vi "UPRcontroller_v00_basedonlsmv66.vi"() -> ()   [LabVIEW 2015] (continued)
                n2507 = property on="srateAODOtt" class="DigNum (strict)"("Visible"=TRUE, "DisabledEnum"=T8."Enabled" ("Disabled")) -> ()  [unwired: 2 in, 2 out]
                n2508 = call "2pparameters.vi"("command"="get") -> ("params out"=w5803:T12)  [unwired: 1 in]
                n2509 = Bundle By Name(cluster=w5803, "type"="Timetrace") -> (w5797:T12)
                n2510 = call "2pparameters.vi"("Params in"=w5797, "command"="set") -> ()  [unwired: 1 out]
                n2511 = property on="Sampling rate" class="DigNum (strict)"("Visible"=FALSE, "DisabledEnum"=T8."Disabled" ("Disabled")) -> ()  [unwired: 2 in, 2 out]
              }
            }
          }
          event "Laserpower  (%)": Value Change {
            n2512 = event-data() -> ("OldVal"=w5832:dbl, "NewVal"=w5833:dbl)  [unwired: 1 in, 4 out]
            n2513 = Not Equal?(x=w5832, y=w5833) -> (x != y?=w5834:bool)
            n2514 = case shown="True" w5834 {
              tunnel: w5833 -> [_ w5836]
              frame False {
              }
              frame True {
                n2515 = local read "wavelength(nm)"() -> (w5837:dbl)
                n2516 = call "configuration.vi"("command"="get") -> ("config out"=w5841:T14)  [unwired: 2 in, 1 out]
                n2517 = call "pockelscellcalibration.vi"("l"=w5837, "T"=w5836) -> ("Vout"=w5835:dbl)
                n2518 = Unbundle By Name(w5841) -> ("Vto2P"=w5840:i32, "AOlines"=w5839:tag[])
                n2519 = property on="lpow" class="DigNum (strict)"("Value"=w5836) -> ()  [unwired: 2 in, 2 out]
                n2520 = local write "Vpockels"(w5835) -> ()
                n2521 = Index Array(array=w5839, index=w5840) -> (element=w5838:tag)
                n2522 = call-poly <vilib>:"DAQmx Create Virtual Channel.vi"("physical channels"=w5838) -> ("task out"=w5844:refnum<k21>, "error out"=w5843:errorcluster)  [unwired: 13 in]
                n2523 = call-poly <vilib>:"DAQmx Write.vi"("task/channels in"=w5844, "data"=w5835, "error in"=w5843) -> ("task out"=w5845:refnum<k21>, "error out"=w5846:errorcluster)  [unwired: 10 in, 1 out]
                n2524 = call <vilib>:"DAQmx Start Task.vi"("task/channels in"=w5845, "error in"=w5846) -> ("task out"=w5847:refnum<k21>, "error out"=w5848:errorcluster)  [unwired: 12 in]
                n2525 = call <vilib>:"DAQmx Stop Task.vi"("task/channels in"=w5847, "error in"=w5848) -> ("task out"=w5849:refnum<k21>, "error out"=w5850:errorcluster)  [unwired: 12 in]
                n2526 = call <vilib>:"DAQmx Clear Task.vi"("task in"=w5849, "error in"=w5850) -> ()  [unwired: 13 in, 1 out]
              }
            }
          }
          event "lpow": Value Change {
            n2527 = event-data() -> ("OldVal"=w5851:dbl, "NewVal"=w5852:dbl)  [unwired: 1 in, 4 out]
            n2528 = Not Equal?(x=w5851, y=w5852) -> (x != y?=w5853:bool)
            n2529 = case shown="True" w5853 {
              tunnel: w5852 -> [_ w5856]
              frame False {
              }
              frame True {
                n2530 = local read "wavelength(nm)"() -> (w5855:dbl)
                n2531 = call "pockelscellcalibration.vi"("l"=w5855, "T"=w5856) -> ("Vout"=w5854:dbl)
                n2532 = call "configuration.vi"("command"="get") -> ("config out"=w5860:T14)  [unwired: 2 in, 1 out]
                n2533 = Unbundle By Name(w5860) -> ("Vto2P"=w5859:i32, "AOlines"=w5858:tag[])
                n2534 = local write "Vpockels"(w5854) -> ()
                n2535 = property on="Laserpower  (%)" class="Slide (strict)"("Value"=w5856) -> ()  [unwired: 2 in, 2 out]
                n2536 = Index Array(array=w5858, index=w5859) -> (element=w5857:tag)
                n2537 = call-poly <vilib>:"DAQmx Create Virtual Channel.vi"("physical channels"=w5857) -> ("task out"=w5863:refnum<k21>, "error out"=w5862:errorcluster)  [unwired: 13 in]
                n2538 = call-poly <vilib>:"DAQmx Write.vi"("task/channels in"=w5863, "data"=w5854, "error in"=w5862) -> ("task out"=w5864:refnum<k21>, "error out"=w5865:errorcluster)  [unwired: 10 in, 1 out]
                n2539 = call <vilib>:"DAQmx Start Task.vi"("task/channels in"=w5864, "error in"=w5865) -> ("task out"=w5866:refnum<k21>, "error out"=w5867:errorcluster)  [unwired: 12 in]
                n2540 = call <vilib>:"DAQmx Stop Task.vi"("task/channels in"=w5866, "error in"=w5867) -> ("task out"=w5868:refnum<k21>, "error out"=w5869:errorcluster)  [unwired: 12 in]
                n2541 = call <vilib>:"DAQmx Clear Task.vi"("task in"=w5868, "error in"=w5869) -> ()  [unwired: 13 in, 1 out]
              }
            }
          }
          event "sealtest": Value Change {
            n2542 = event-data() -> ()  [unwired: 1 in, 6 out]
            n2543 = case shown="True" "sealtest" {
              frame False {
              }
              frame True {
                n2544 = stacked-sequence {
                  seq-local: [w5871 _ _ _ _ _ _] -> [_ w5906 _ w5958 _ _ _]
                  frame #0 {
                    n2545 = stacked-sequence {
                      tunnel: [_ w5885 _] -> w5871
                      frame #0 {
                        n2546 = call "2pparameters.vi"("command"="get") -> ("params out"=w5877:T12)  [unwired: 1 in]
                        n2547 = Unbundle By Name(w5877) -> ("autoshutter"=w5878:bool, "aAS"=w5872:u32[])
                        n2548 = local read "OCchecked?"() -> (w5875:bool)
                        n2549 = call "sealtestwfparams.vi"("command"="set") -> ()  [unwired: 6 in, 1 out]
                        n2550 = case shown="False" w5875 {
                          frame False {
                            n2551 = One Button Dialog(message="Is the OC gain correct?", button name ("OK")="ok") -> (true=w5879:bool)
                            n2552 = local write "OCchecked?"(w5879) -> ()
                          }
                          frame True {
                          }
                        }
                        n2553 = case shown="True" w5878 {
                          tunnel: w5872 -> [_ w5882]
                          frame False {
                          }
                          frame True {
                            n2554 = call "shuttercontrol_multi.vi"("Autoshutter Chans"=w5882, "command"="close") -> ()  [unwired: 1 in, 1 out]
                          }
                        }
                        n2555 = call "allAI-temp.vi"("command"=enum16{"get", "set", "clear", "append"}."clear") -> ()  [unwired: 3 in, 2 out]
                      }
                      frame #1 {
                        n2556 = call "sealtestwfparams.vi"("command"="get") -> ("Params out"=w5891:T25)  [unwired: 6 in]
                        n2557 = Unbundle By Name(w5891) -> ("AO parameters"=w5889:T26)
                        n2558 = Index Array(array=w5889, index=0) -> (element=w5888:T27)
                        n2559 = call "generateRampedSquareWave_fromAOparameters.vi"("AO params"=w5888) -> ("Waveform"=w5884:waveform(dbl), "wflength"=w5885:i32)
                        n2560 = Build Array(w5884) -> (w5887:waveform(dbl)[])
                        n2561 = call "waveformssealtestbuffer.vi"("AO wf in"=w5887, "command"="set") -> ()  [unwired: 1 out]
                      }
                      frame #2 {
                        n2562 = local read "Vholding (mV)"() -> (w5894:sgl)
                        n2563 = local read "Current Clamp"() -> (w5900:bool)
                        n2564 = local read "Voltage Clamp"() -> (w5899:bool)
                        n2565 = local read "OCgain"() -> (w5895:sgl)
                        n2566 = local read "CC_ICgain"() -> (w5898:dbl)
                        n2567 = local read "holdon"() -> (w5893:bool)
                        n2568 = call "patchparameters.vi"("command"="get") -> ("Params out"=w5902:T16)  [unwired: 1 in]
                        n2569 = Bundle By Name(cluster=w5902, "VC"=w5899, "CC"=w5900, "CC_icg (pA/mv)"=w5898, "VC_icg (mV/mV)"=10.0, "OCG (mV/pA)"=w5895, "OVG (mV/mV)"=0.1, "Vhold (mV)"=w5894, "holdon"=w5893) -> (w5901:T16)
                        n2570 = call "patchparameters.vi"("Params in"=w5901, "command"="set") -> ()  [unwired: 1 out]
                      }
                    }
                  }
                  frame #1 {
                    w5905 = 2
                    n2571 = call "patchparameters.vi"("command"="get") -> ("Params out"=w5913:T16)  [unwired: 1 in]
                    n2572 = Unbundle By Name(w5913) -> ("holdon"=w5912:bool, "Vhold (mV)"=w5911:sgl, "CC_icg (pA/mv)"=w5919:sgl, "CC"=w5917:bool, "VC_icg (mV/mV)"=w5918:sgl)
                    n2573 = Select(t=w5919, s=w5917, f=w5918) -> (s? t:f=w5920:sgl)
                    n2574 = To Single Precision Float(number=0.001 ("y")) -> (single precision float=w5921:sgl)
                    n2575 = Compound Arithmetic op=MULTIPLY(w5911, w5920, w5921) -> (w5915:sgl)
                    n2576 = case shown="False" w5912 {
                      tunnel: w5915 -> [_ w5933]
                      tunnel: [0.0 w5933] -> w5908
                      frame False {
                      }
                      frame True {
                      }
                    }
                    n2577 = Greater Than 0?(x=w5905) -> (x > 0?=w5907:bool)
                    n2578 = case shown="True" w5907 {
                      tunnel: w5906 -> [_ w5922]
                      tunnel: w5905 -> [_ w5925]
                      frame False {
                      }
                      frame True {
                        n2579 = Initialize Array(sgl 0.0 ("element"), w5925, w5922) -> (w5923:sgl[][])
                        n2580 = call "allAI-temp.vi"("array in"=w5923, "command"=enum16{"get", "set", "clear", "append"}."set") -> ()  [unwired: 2 in, 2 out]
                      }
                    }
                    n2581 = flat-sequence {
                      tunnel: w5906 -> [w5929]
                      tunnel: w5906 -> [w5928]
                      tunnel: [w5928] -> w5910
                      tunnel: [w5927] -> w5909
                      tunnel: w5908 -> [w5927]
                      tunnel: w5910 -> [w5931]
                      tunnel: w5909 -> [w5930]
                      frame #0 {
                        n2582 = call "prepAI_sealtest.vi"("samples per channel"=w5929) -> ()  [unwired: 2 in]
                      }
                      frame #1 {
                        n2583 = call "prepAO_sealtest.vi"("Vhold"=w5930, "samples per channel"=w5931) -> ()  [unwired: 1 in]
                      }
                    }
                  }
                  frame #2 {
                    n2584 = stacked-sequence {
                      frame #0 {
                        n2585 = call "tempconfigAO_seal.vi"("command"="get") -> ("Temp Config out"=w5937:T28)  [unwired: 1 in]
                        n2586 = Unbundle By Name(w5937) -> ("AO"=w5938:refnum<k21>[], "E_AO"=w5939:errorcluster[])
                        n2587 = for {
                          tunnel: w5938 -> [w5947] mode=indexing
                          tunnel: w5939 -> [w5946] mode=indexing
                          tunnel: [w5945] -> w5941 mode=indexing
                          tunnel: [w5944] -> w5942 mode=indexing
                          n2588 = call <vilib>:"DAQmx Start Task.vi"("task/channels in"=w5947, "error in"=w5946) -> ("task out"=w5945:refnum<k21>, "error out"=w5944:errorcluster)  [unwired: 12 in]
                        }
                        n2589 = call "tempconfigAO_seal.vi"("command"="get") -> ("Temp Config out"=w5940:T28)  [unwired: 1 in]
                        n2590 = Bundle By Name(cluster=w5940, "AO"=w5941, "E_AO"=w5942) -> (w5943:T28)
                        n2591 = call "tempconfigAO_seal.vi"("Temp Config in"=w5943, "command"="set") -> ()  [unwired: 1 out]
                      }
                      frame #1 {
                        n2592 = call "tempconfigAI_seal.vi"("command"="get") -> ("Temp Config out"=w5949:T29)  [unwired: 1 in]
                        n2593 = Unbundle By Name(w5949) -> ("AI"=w5954:refnum<k21>, "E_AI"=w5955:errorcluster)
                        n2594 = call <vilib>:"DAQmx Start Task.vi"("task/channels in"=w5954, "error in"=w5955) -> ("task out"=w5956:refnum<k21>, "error out"=w5957:errorcluster)  [unwired: 12 in]
                        n2595 = call "tempconfigAI_seal.vi"("command"="get") -> ("Temp Config out"=w5951:T29)  [unwired: 1 in]
                        n2596 = Bundle By Name(cluster=w5951, "AI"=w5956, "E_AI"=w5957) -> (w5953:T29)
                        n2597 = call "tempconfigAI_seal.vi"("Temp Config in"=w5953, "command"="set") -> ()  [unwired: 1 out]
                      }
                    }
                  }
                  frame #3 {
                    n2598 = while {
                      tunnel: w5958 -> [w5959]
                      stop <- w5960 stop-if-true
                      n2599 = stacked-sequence {
                        seq-local: [_ _ _ w6001 _ _] -> [_ _ _ _ w6053 _]
                        seq-local: [w5962 _ _ _ _ _] -> [_ w5971 _ w5994 w6042 w6073]
                        tunnel: w5959 -> [_ _ w5979 _ w6041 _]
                        frame #0 {
                          n2600 = call "patchparameters.vi"("command"="get") -> ("Params out"=w5969:T16)  [unwired: 1 in]
                          n2601 = local read "Vholding (mV)"() -> (w5966:sgl)
                          n2602 = Unbundle By Name(w5969) -> ("Vhold (mV)"=w5965:sgl, "holdon"=w5968:bool)
                          n2603 = local read "holdon"() -> (w5967:bool)
                          n2604 = Not Equal?(x=w5966, y=w5965) -> (x != y?=w5964:bool)
                          n2605 = Not Equal?(x=w5968, y=w5967) -> (x != y?=w5963:bool)
                          n2606 = Or(x=w5964, y=w5963) -> (x .or. y?=w5962:bool)
                        }
                        frame #1 {
                          n2607 = case shown="True" w5971 {
                            frame False {
                            }
                            frame True {
                              n2608 = local read "Vholding (mV)"() -> (w5974:sgl)
                              n2609 = local read "holdon"() -> (w5972:bool)
                              n2610 = call "patchparameters.vi"("command"="get") -> ("Params out"=w5975:T16)  [unwired: 1 in]
                              n2611 = Bundle By Name(cluster=w5975, "Vhold (mV)"=w5974, "holdon"=w5972) -> (w5973:T16)
                              n2612 = call "patchparameters.vi"("Params in"=w5973, "command"="set") -> ()  [unwired: 1 out]
                            }
                          }
                        }
                        frame #2 {
                          n2613 = call "tempconfigAI_seal.vi"("command"="get") -> ("Temp Config out"=w5989:T29)  [unwired: 1 in]
                          n2614 = Unbundle By Name(w5989) -> ("AI"=w5988:refnum<k21>, "E_AI"=w5987:errorcluster)
                          n2615 = call-poly <vilib>:"DAQmx Read.vi"("task/channels in"=w5988, "number of samples per channel"=w5979, "timeout"=10.0, "error in"=w5987) -> ("task out"=w5983:refnum<k21>, "data"=w5980:i16[][], "error out"=w5992:errorcluster)  [unwired: 9 in]
                          n2616 = call "tempconfigAI_seal.vi"("command"="get") -> ("Temp Config out"=w5984:T29)  [unwired: 1 in]
                          n2617 = Bundle By Name(cluster=w5984, "AI"=w5983, "E_AI"=w5992) -> (w5991:T29)
                          n2618 = To Single Precision Float(number=w5980) -> (single precision float=w5982:sgl[][])
                          n2619 = call "tempconfigAI_seal.vi"("Temp Config in"=w5991, "command"="set") -> ()  [unwired: 1 out]
                          n2620 = call "allAI-temp.vi"("array in"=w5982, "command"=enum16{"get", "set", "clear", "append"}."set") -> ()  [unwired: 2 in, 2 out]
                        }
                        frame #3 {
                          n2621 = case shown="True" w5994 {
                            frame False {
                            }
                            frame True {
                              n2622 = call "tempconfigAO_seal.vi"("command"="get") -> ("Temp Config out"=w6030:T28)  [unwired: 1 in]
                              n2623 = Unbundle By Name(w6030) -> ("AO"=w6029:refnum<k21>[], "E_AO"=w6028:errorcluster[])
                              n2624 = call "tempconfigAI_seal.vi"("command"="get") -> ("Temp Config out"=w6017:T29)  [unwired: 1 in]
                              n2625 = Unbundle By Name(w6017) -> ("AI"=w6018:refnum<k21>, "E_AI"=w6019:errorcluster)
                              n2626 = for {
                                tunnel: w6029 -> [w6034] mode=indexing
                                tunnel: w6028 -> [w6033] mode=indexing
                                tunnel: [w6032] -> w6024 mode=indexing
                                n2627 = call <vilib>:"DAQmx Stop Task.vi"("task/channels in"=w6034, "error in"=w6033) -> ("task out"=w6035:refnum<k21>, "error out"=w6036:errorcluster)  [unwired: 12 in]
                                n2628 = call <vilib>:"DAQmx Clear Task.vi"("task in"=w6035, "error in"=w6036) -> ("error out"=w6032:errorcluster)  [unwired: 13 in]
                              }
                              n2629 = call <vilib>:"DAQmx Stop Task.vi"("task/channels in"=w6018, "error in"=w6019) -> ("task out"=w6015:refnum<k21>, "error out"=w6014:errorcluster)  [unwired: 12 in]
                              n2630 = call <vilib>:"DAQmx Clear Task.vi"("task in"=w6015, "error in"=w6014) -> ("error out"=w6013:errorcluster)  [unwired: 13 in]
                              n2631 = call "tempconfigAO_seal.vi"("command"="get") -> ("Temp Config out"=w6025:T28)  [unwired: 1 in]
                              n2632 = Bundle By Name(cluster=w6025, "E_AO"=w6024) -> (w6023:T28)
                              n2633 = call "tempconfigAI_seal.vi"("command"="get") -> ("Temp Config out"=w6021:T29)  [unwired: 1 in]
                              n2634 = Bundle By Name(cluster=w6021, "E_AI"=w6013) -> (w6012:T29)
                              n2635 = call "tempconfigAO_seal.vi"("Temp Config in"=w6023, "command"="set") -> ()  [unwired: 1 out]
                              n2636 = call "tempconfigAI_seal.vi"("Temp Config in"=w6012, "command"="set") -> ()  [unwired: 1 out]
                            }
                          }
                          n2637 = call "allAI-temp.vi"("command"=enum16{"get", "set", "clear", "append"}."get") -> ("array out"=w5998:sgl[][])  [unwired: 3 in, 1 out]
                          n2638 = call "tempconfigAI_seal.vi"("command"="get") -> ("Temp Config out"=w6010:T29)  [unwired: 1 in]
                          n2639 = Unbundle By Name(w6010) -> ("header"=w5993:dbl[])
                          n2640 = Index Array(array=w5998, index (row) #1=1 ("index (row)"), index (row) #2=0 ("index (row)")) -> (element #1=w5996:sgl[], element #2=w5995:sgl[])  [unwired: 2 in]
                          n2641 = local read "OCgain"() -> (w6003:sgl)
                          n2642 = call "Unscaledtoscaled.vi"("Unscaled Data"=w5996, "Header Information"=w5993) -> ("Array"=w6008:sgl[])  [unwired: 1 in]
                          n2643 = call "Unscaledtoscaled.vi"("Unscaled Data"=w5995, "Header Information"=w5993) -> ("Array"=w6011:sgl[])  [unwired: 1 in]
                          n2644 = Multiply(x=w6008, y=0.1) -> (x*y=w6005:dbl[])
                          n2645 = Divide(x=w6011, y=w6003) -> (x/y=w6004:sgl[])
                          n2646 = Build Array(w6005, w6004) -> (w6007:dbl[][])
                          n2647 = Multiply(x=w6007, y=1000.0) -> (x*y=w6001:dbl[][])
                          "Patch readout" <- w6001
                        }
                        frame #4 {
                          n2648 = case shown="True" w6042 {
                            tunnel: w6041 -> [_ w6054]
                            frame False {
                            }
                            frame True {
                              n2649 = call "patchparameters.vi"("command"="get") -> ("Params out"=w6058:T16)  [unwired: 1 in]
                              n2650 = Unbundle By Name(w6058) -> ("holdon"=w6057:bool, "Vhold (mV)"=w6056:sgl, "CC_icg (pA/mv)"=w6064:sgl, "CC"=w6062:bool, "VC_icg (mV/mV)"=w6063:sgl)
                              n2651 = Select(t=w6064, s=w6062, f=w6063) -> (s? t:f=w6065:sgl)
                              n2652 = To Single Precision Float(number=0.001 ("y")) -> (single precision float=w6066:sgl)
                              n2653 = Compound Arithmetic op=MULTIPLY(w6056, w6065, w6066) -> (w6060:sgl)
                              n2654 = case shown="True" w6057 {
                                tunnel: w6060 -> [_ w6071]
                                tunnel: [0.0 w6071] -> w6055
                                frame False {
                                }
                                frame True {
                                }
                              }
                              n2655 = flat-sequence {
                                tunnel: w6054 -> [w6067]
                                tunnel: w6055 -> [w6069]
                                tunnel: w6054 -> [w6068]
                                frame #0 {
                                n2656 = call "prepAI_sealtest.vi"("samples per channel"=w6067) -> ()  [unwired: 2 in]
                                }
                                frame #1 {
                                n2657 = call "prepAO_sealtest.vi"("Vhold"=w6069, "samples per channel"=w6068) -> ()  [unwired: 1 in]
                                }
                              }
                            }
                          }
                          n2658 = call "sealtestwfparams.vi"("command"="get") -> ("Params out"=w6047:T25)  [unwired: 6 in]
                          n2659 = Unbundle By Name(w6047) -> ("AO parameters"=w6048:T26)
                          n2660 = Index Array(array=w6048, index=0) -> (element=w6050:T27)
                          n2661 = Unbundle By Name(w6050) -> ("Cycles"=w6045:dbl, "Start amplitude (V)"=w6044:dbl, "Sampling frequency (Hz)"=w6043:dbl)
                          n2662 = local read "fitpoints"() -> (w6051:dbl)
                          n2663 = script code="V=data(1,:);\nI=data(2,:);\ntres=mean(V);\nspc=(nsamp./ncyc);\nV=V(spc+1:end-spc);\nI=I(spc+1:end-spc);\ndV=mean(V(V>tres))-mean(V(V<tres))\nIcyc=reshape(I,[spc ncyc-2]);\nIcyc=Icyc';\nIcyc=mean(Icyc,1);\ndIss=mean(Icyc(floor(spc*0.15):floor(spc/2)-2))-mean(Icyc(spc*0.65:spc-2))\nRm=dV*1e3/dIss;\n[maxi,ind]=max(Icyc);\nIfit=Icyc(ind+1:ind+1+points-1)-0.5*(mean(Icyc(floor(spc*0.15):floor(spc/2)-2))+mean(Icyc(spc*0.65:spc-2)))\nt=(3:points-1+3)./srate*1000;\nt=t';\nIfit=Ifit';\nc=fit(t,Ifit, 'exp1');\ncoeffs=coeffvalues(c);\nIa=coeffs(1);\nRa=dV*1e3./Ia/2;\ntau=-1./coeffs(2);\ncap=tau/Ra*1000;"("data"=w6053, "nsamp"=w6041, "ncyc"=w6045, "maxV"=w6044, "points"=w6051, "srate"=w6043) -> ("cap"=w6040:dbl, "Ra"=w6039:dbl, "Icyc"=w6038:dbl[], "Rm"=w6037:dbl)  [unwired: 1 in, 1 out]
                          n2664 = local read "set as Rp?"() -> (w6052:bool)
                          n2665 = local write "Cmembrane"(w6040) -> ()
                          n2666 = local write "Rmembrane (MOhm)"(w6037) -> ()
                          n2667 = local write "Racces (MOhm)"(w6039) -> ()
                          n2668 = case shown="True" w6052 {
                            tunnel: w6037 -> [_ w6072]
                            frame False {
                            }
                            frame True {
                              n2669 = local write "Rpipette (MOhm)"(w6072) -> ()
                            }
                          }
                          n2670 = local write "Ifit"(w6038) -> ()
                        }
                        frame #5 {
                          n2671 = local read "set as Rp?"() -> (w6074:bool)
                          n2672 = case shown="True" w6073 {
                            frame False {
                            }
                            frame True {
                              n2673 = stacked-sequence {
                                frame #0 {
                                n2674 = call "tempconfigAO_seal.vi"("command"="get") -> ("Temp Config out"=w6081:T28)  [unwired: 1 in]
                                n2675 = Unbundle By Name(w6081) -> ("AO"=w6080:refnum<k21>[], "E_AO"=w6079:errorcluster[])
                                n2676 = for {
                                tunnel: w6080 -> [w6088] mode=indexing
                                tunnel: w6079 -> [w6087] mode=indexing
                                tunnel: [w6086] -> w6077 mode=indexing
                                tunnel: [w6085] -> w6076 mode=indexing
                                n2677 = call <vilib>:"DAQmx Start Task.vi"("task/channels in"=w6088, "error in"=w6087) -> ("task out"=w6086:refnum<k21>, "error out"=w6085:errorcluster)  [unwired: 12 in]
                                }
                                n2678 = call "tempconfigAO_seal.vi"("command"="get") -> ("Temp Config out"=w6078:T28)  [unwired: 1 in]
                                n2679 = Bundle By Name(cluster=w6078, "AO"=w6077, "E_AO"=w6076) -> (w6075:T28)
                                n2680 = call "tempconfigAO_seal.vi"("Temp Config in"=w6075, "command"="set") -> ()  [unwired: 1 out]
                                }
                                frame #1 {
                                n2681 = call "tempconfigAI_seal.vi"("command"="get") -> ("Temp Config out"=w6090:T29)  [unwired: 1 in]
                                n2682 = Unbundle By Name(w6090) -> ("AI"=w6095:refnum<k21>, "E_AI"=w6096:errorcluster)
                                n2683 = call <vilib>:"DAQmx Start Task.vi"("task/channels in"=w6095, "error in"=w6096) -> ("task out"=w6097:refnum<k21>, "error out"=w6098:errorcluster)  [unwired: 12 in]
                                n2684 = call "tempconfigAI_seal.vi"("command"="get") -> ("Temp Config out"=w6092:T29)  [unwired: 1 in]
                                n2685 = Bundle By Name(cluster=w6092, "AI"=w6097, "E_AI"=w6098) -> (w6094:T29)
                                n2686 = call "tempconfigAI_seal.vi"("Temp Config in"=w6094, "command"="set") -> ()  [unwired: 1 out]
                                }
                              }
                            }
                          }
                          n2687 = case shown="True" w6074 {
                            frame False {
                            }
                            frame True {
                              n2688 = local write "set as Rp?"(FALSE ("set as Rp?")) -> ()
                            }
                          }
                        }
                      }
                      n2689 = local read "sealtest"() -> (w5961:bool)
                      n2690 = Not(x=w5961) -> (.not. x?=w5960:bool)
                    }
                  }
                  frame #4 {
                    n2691 = call "tempconfigAO_seal.vi"("command"="get") -> ("Temp Config out"=w6125:T28)  [unwired: 1 in]
                    n2692 = Unbundle By Name(w6125) -> ("AO"=w6124:refnum<k21>[], "E_AO"=w6123:errorcluster[])
                    n2693 = call "tempconfigAI_seal.vi"("command"="get") -> ("Temp Config out"=w6112:T29)  [unwired: 1 in]
                    n2694 = call "configuration.vi"("command"="get") -> ("config out"=w6106:T14)  [unwired: 2 in, 1 out]
                    n2695 = Unbundle By Name(w6112) -> ("AI"=w6113:refnum<k21>, "E_AI"=w6114:errorcluster)
                    n2696 = Unbundle By Name(w6106) -> ("Device 1 sampleclock out"=w6103:tag, "Device 1 Starttrigger out"=w6102:tag)
                    n2697 = for {
                      tunnel: w6124 -> [w6129] mode=indexing
                      tunnel: w6123 -> [w6128] mode=indexing
                      tunnel: [w6127] -> w6119 mode=indexing
                      n2698 = call <vilib>:"DAQmx Stop Task.vi"("task/channels in"=w6129, "error in"=w6128) -> ("task out"=w6130:refnum<k21>, "error out"=w6131:errorcluster)  [unwired: 12 in]
                      n2699 = call <vilib>:"DAQmx Clear Task.vi"("task in"=w6130, "error in"=w6131) -> ("error out"=w6127:errorcluster)  [unwired: 13 in]
                    }
                    n2700 = call <vilib>:"DAQmx Stop Task.vi"("task/channels in"=w6113, "error in"=w6114) -> ("task out"=w6110:refnum<k21>, "error out"=w6109:errorcluster)  [unwired: 12 in]
                    n2701 = call <vilib>:"DAQmx Disconnect Terminals.vi"("source terminal"=tag "/Dev1/ai/SampleClock", "destination terminal"=w6103) -> ("error out"=w6100:errorcluster)  [unwired: 13 in]
                    n2702 = call <vilib>:"DAQmx Clear Task.vi"("task in"=w6110, "error in"=w6109) -> ("error out"=w6108:errorcluster)  [unwired: 13 in]
                    n2703 = call "tempconfigAO_seal.vi"("command"="get") -> ("Temp Config out"=w6120:T28)  [unwired: 1 in]
                    n2704 = Bundle By Name(cluster=w6120, "E_AO"=w6119) -> (w6118:T28)
                    n2705 = call "tempconfigAI_seal.vi"("command"="get") -> ("Temp Config out"=w6116:T29)  [unwired: 1 in]
                    n2706 = Bundle By Name(cluster=w6116, "E_AI"=w6108) -> (w6107:T29)
                    n2707 = call "tempconfigAO_seal.vi"("Temp Config in"=w6118, "command"="set") -> ()  [unwired: 1 out]
                    n2708 = call "tempconfigAI_seal.vi"("Temp Config in"=w6107, "command"="set") -> ()  [unwired: 1 out]
                    n2709 = call <vilib>:"DAQmx Disconnect Terminals.vi"("source terminal"=tag "/Dev1/ai/StartTrigger", "destination terminal"=w6102, "error in"=w6100) -> ()  [unwired: 12 in, 1 out]
                  }
                  frame #5 {
                    n2710 = call "zeropatch.vi"() -> ()  [unwired: 12 in]
                  }
                  frame #6 {
                    w6135 = T24 4 items=["no dialog", "OK message", "continue or stop message", "OK message + warnings", "continue/stop + warnings"] ("type of dialog (OK msg:1)")
                    n2711 = call "displayerrors.vi"() -> ("error IO"=w6134:errorcluster)
                    n2712 = call <vilib>:"Simple Error Handler.vi"("type of dialog (OK msg:1)"=w6135, "error in (no error)"=w6134) -> ("error out"=w6133:errorcluster)  [unwired: 3 in, 4 out]
                    n2713 = call <vilib>:"Clear Errors.vi"("error in (no error)"=w6133) -> ("error out"=w6132:errorcluster)  [unwired: 5 in, 1 out]
                    n2714 = call "seterrors.vi"("error IO"=w6132) -> ()
                  }
                }
              }
            }
          }
          event "readpatch": Value Change {
            n2715 = event-data() -> ()  [unwired: 1 in, 6 out]
            n2716 = local read "readpatch"() -> (w6136:bool)
            n2717 = case shown="True" w6136 {
              frame False {
              }
              frame True {
                n2718 = stacked-sequence {
                  seq-local: [w6137 _ _ _ _ _] -> [_ w6172 _ w6224 _ _]
                  frame #0 {
                    n2719 = stacked-sequence {
                      tunnel: [_ w6151 _] -> w6137
                      frame #0 {
                        n2720 = call "2pparameters.vi"("command"="get") -> ("params out"=w6143:T12)  [unwired: 1 in]
                        n2721 = Unbundle By Name(w6143) -> ("autoshutter"=w6144:bool, "aAS"=w6138:u32[])
                        n2722 = local read "OCchecked?"() -> (w6141:bool)
                        n2723 = call "sealtestwfparams.vi"("command"="set") -> ()  [unwired: 6 in, 1 out]
                        n2724 = case shown="False" w6141 {
                          frame False {
                            n2725 = One Button Dialog(message="Is the OC gain correct?", button name ("OK")="ok") -> (true=w6145:bool)
                            n2726 = local write "OCchecked?"(w6145) -> ()
                          }
                          frame True {
                          }
                        }
                        n2727 = case shown="True" w6144 {
                          tunnel: w6138 -> [_ w6148]
                          frame False {
                          }
                          frame True {
                            n2728 = call "shuttercontrol_multi.vi"("Autoshutter Chans"=w6148, "command"="close") -> ()  [unwired: 1 in, 1 out]
                          }
                        }
                        n2729 = call "allAI-temp.vi"("command"=enum16{"get", "set", "clear", "append"}."clear") -> ()  [unwired: 3 in, 2 out]
                      }
                      frame #1 {
                        n2730 = call "sealtestwfparams.vi"("command"="get") -> ("Params out"=w6157:T25)  [unwired: 6 in]
                        n2731 = Unbundle By Name(w6157) -> ("AO parameters"=w6155:T26)
                        n2732 = Index Array(array=w6155, index=1) -> (element=w6154:T27)
                        n2733 = call "generateRampedSquareWave_fromAOparameters.vi"("AO params"=w6154) -> ("Waveform"=w6150:waveform(dbl), "wflength"=w6151:i32)
                        n2734 = Build Array(w6150) -> (w6153:waveform(dbl)[])
                        n2735 = call "waveformssealtestbuffer.vi"("AO wf in"=w6153, "command"="set") -> ()  [unwired: 1 out]
                      }
                      frame #2 {
                        n2736 = local read "Vholding (mV)"() -> (w6160:sgl)
                        n2737 = local read "Current Clamp"() -> (w6166:bool)
                        n2738 = local read "Voltage Clamp"() -> (w6165:bool)
                        n2739 = local read "OCgain"() -> (w6161:sgl)
                        n2740 = local read "CC_ICgain"() -> (w6164:dbl)
                        n2741 = local read "holdon"() -> (w6159:bool)
                        n2742 = call "patchparameters.vi"("command"="get") -> ("Params out"=w6168:T16)  [unwired: 1 in]
                        n2743 = Bundle By Name(cluster=w6168, "VC"=w6165, "CC"=w6166, "CC_icg (pA/mv)"=w6164, "VC_icg (mV/mV)"=10.0, "OCG (mV/pA)"=w6161, "OVG (mV/mV)"=0.1, "Vhold (mV)"=w6160, "holdon"=w6159) -> (w6167:T16)
                        n2744 = call "patchparameters.vi"("Params in"=w6167, "command"="set") -> ()  [unwired: 1 out]
                      }
                    }
                  }
                  frame #1 {
                    w6171 = 2
                    n2745 = call "patchparameters.vi"("command"="get") -> ("Params out"=w6179:T16)  [unwired: 1 in]
                    n2746 = Unbundle By Name(w6179) -> ("holdon"=w6178:bool, "Vhold (mV)"=w6177:sgl, "CC_icg (pA/mv)"=w6185:sgl, "CC"=w6183:bool, "VC_icg (mV/mV)"=w6184:sgl)
                    n2747 = Select(t=w6185, s=w6183, f=w6184) -> (s? t:f=w6186:sgl)
                    n2748 = To Single Precision Float(number=0.001 ("y")) -> (single precision float=w6187:sgl)
                    n2749 = Compound Arithmetic op=MULTIPLY(w6177, w6186, w6187) -> (w6181:sgl)
                    n2750 = case shown="False" w6178 {
                      tunnel: w6181 -> [_ w6199]
                      tunnel: [0.0 w6199] -> w6174
                      frame False {
                      }
                      frame True {
                      }
                    }
                    n2751 = Greater Than 0?(x=w6171) -> (x > 0?=w6173:bool)
                    n2752 = case shown="True" w6173 {
                      tunnel: w6172 -> [_ w6188]
                      tunnel: w6171 -> [_ w6191]
                      frame False {
                      }
                      frame True {
                        n2753 = Initialize Array(sgl 0.0 ("element"), w6191, w6188) -> (w6189:sgl[][])
                        n2754 = call "allAI-temp.vi"("array in"=w6189, "command"=enum16{"get", "set", "clear", "append"}."set") -> ()  [unwired: 2 in, 2 out]
                      }
                    }
                    n2755 = flat-sequence {
                      tunnel: w6172 -> [w6195]
                      tunnel: w6172 -> [w6194]
                      tunnel: [w6194] -> w6176
                      tunnel: [w6193] -> w6175
                      tunnel: w6174 -> [w6193]
                      tunnel: w6176 -> [w6197]
                      tunnel: w6175 -> [w6196]
                      frame #0 {
                        n2756 = call "prepAI_sealtest.vi"("samples per channel"=w6195) -> ()  [unwired: 2 in]
                      }
                      frame #1 {
                        n2757 = call "prepAO_sealtest.vi"("Vhold"=w6196, "samples per channel"=w6197) -> ()  [unwired: 1 in]
                      }
                    }
                  }
                  frame #2 {
                    n2758 = stacked-sequence {
                      frame #0 {
                        n2759 = call "tempconfigAO.vi"("command"="get") -> ("Temp Config out"=w6203:T28)  [unwired: 1 in]
                        n2760 = Unbundle By Name(w6203) -> ("AO"=w6204:refnum<k21>[], "E_AO"=w6205:errorcluster[])
                        n2761 = for {
                          tunnel: w6204 -> [w6213] mode=indexing
                          tunnel: w6205 -> [w6212] mode=indexing
                          tunnel: [w6211] -> w6207 mode=indexing
                          tunnel: [w6210] -> w6208 mode=indexing
                          n2762 = call <vilib>:"DAQmx Start Task.vi"("task/channels in"=w6213, "error in"=w6212) -> ("task out"=w6211:refnum<k21>, "error out"=w6210:errorcluster)  [unwired: 12 in]
                        }
                        n2763 = call "tempconfigAO.vi"("command"="get") -> ("Temp Config out"=w6206:T28)  [unwired: 1 in]
                        n2764 = Bundle By Name(cluster=w6206, "AO"=w6207, "E_AO"=w6208) -> (w6209:T28)
                        n2765 = call "tempconfigAO.vi"("Temp Config in"=w6209, "command"="set") -> ()  [unwired: 1 out]
                      }
                      frame #1 {
                        n2766 = call "tempconfigAI.vi"("command"="get") -> ("Temp Config out"=w6215:T29)  [unwired: 1 in]
                        n2767 = Unbundle By Name(w6215) -> ("AI"=w6220:refnum<k21>, "E_AI"=w6221:errorcluster)
                        n2768 = call <vilib>:"DAQmx Start Task.vi"("task/channels in"=w6220, "error in"=w6221) -> ("task out"=w6222:refnum<k21>, "error out"=w6223:errorcluster)  [unwired: 12 in]
                        n2769 = call "tempconfigAI.vi"("command"="get") -> ("Temp Config out"=w6217:T29)  [unwired: 1 in]
                        n2770 = Bundle By Name(cluster=w6217, "AI"=w6222, "E_AI"=w6223) -> (w6219:T29)
                        n2771 = call "tempconfigAI.vi"("Temp Config in"=w6219, "command"="set") -> ()  [unwired: 1 out]
                      }
                    }
                  }
                  frame #3 {
                    n2772 = while {
                      tunnel: w6224 -> [w6225]
                      stop <- w6226 stop-if-true
                      n2773 = local read "readpatch"() -> (w6229:bool)
                      n2774 = Not(x=w6229) -> (.not. x?=w6228:bool)
                      n2775 = case shown="False" w6228 {
                        tunnel: w6225 -> [w6230 _]
                        frame False {
                          n2776 = stacked-sequence {
                            seq-local: [w6231 _ _ _ _ _] -> [_ w6240 _ w6263 w6310 w6329]
                            tunnel: w6230 -> [_ _ w6248 _ w6309 _]
                            frame #0 {
                              n2777 = call "patchparameters.vi"("command"="get") -> ("Params out"=w6238:T16)  [unwired: 1 in]
                              n2778 = local read "Vholding (mV)"() -> (w6235:sgl)
                              n2779 = Unbundle By Name(w6238) -> ("Vhold (mV)"=w6234:sgl, "holdon"=w6237:bool)
                              n2780 = local read "holdon"() -> (w6236:bool)
                              n2781 = Not Equal?(x=w6235, y=w6234) -> (x != y?=w6233:bool)
                              n2782 = Not Equal?(x=w6237, y=w6236) -> (x != y?=w6232:bool)
                              n2783 = Or(x=w6233, y=w6232) -> (x .or. y?=w6231:bool)
                            }
                            frame #1 {
                              n2784 = case shown="False" w6240 {
                                frame False {
                                }
                                frame True {
                                n2785 = local read "Vholding (mV)"() -> (w6243:sgl)
                                n2786 = local read "holdon"() -> (w6241:bool)
                                n2787 = call "patchparameters.vi"("command"="get") -> ("Params out"=w6244:T16)  [unwired: 1 in]
                                n2788 = Bundle By Name(cluster=w6244, "Vhold (mV)"=w6243, "holdon"=w6241) -> (w6242:T16)
                                n2789 = call "patchparameters.vi"("Params in"=w6242, "command"="set") -> ()  [unwired: 1 out]
                                }
                              }
                            }
                            frame #2 {
                              n2790 = call "tempconfigAI.vi"("command"="get") -> ("Temp Config out"=w6258:T29)  [unwired: 1 in]
                              n2791 = Unbundle By Name(w6258) -> ("AI"=w6257:refnum<k21>, "E_AI"=w6256:errorcluster)
                              n2792 = call-poly <vilib>:"DAQmx Read.vi"("task/channels in"=w6257, "number of samples per channel"=w6248, "timeout"=10.0, "error in"=w6256) -> ("task out"=w6252:refnum<k21>, "data"=w6249:i16[][], "error out"=w6261:errorcluster)  [unwired: 9 in]
                              n2793 = call "tempconfigAI.vi"("command"="get") -> ("Temp Config out"=w6253:T29)  [unwired: 1 in]
                              n2794 = Bundle By Name(cluster=w6253, "AI"=w6252, "E_AI"=w6261) -> (w6260:T29)
                              n2795 = To Single Precision Float(number=w6249) -> (single precision float=w6251:sgl[][])
                              n2796 = call "tempconfigAI.vi"("Temp Config in"=w6260, "command"="set") -> ()  [unwired: 1 out]
                              n2797 = call "allAI-temp.vi"("array in"=w6251, "command"=enum16{"get", "set", "clear", "append"}."set") -> ()  [unwired: 2 in, 2 out]
                            }
                            frame #3 {
                              n2798 = case shown="True" w6263 {
                                frame False {
                                }
                                frame True {
                                n2799 = call "tempconfigAO.vi"("command"="get") -> ("Temp Config out"=w6302:T28)  [unwired: 1 in]
                                n2800 = Unbundle By Name(w6302) -> ("AO"=w6301:refnum<k21>[], "E_AO"=w6300:errorcluster[])
                                n2801 = call "tempconfigAI.vi"("command"="get") -> ("Temp Config out"=w6289:T29)  [unwired: 1 in]
                                n2802 = Unbundle By Name(w6289) -> ("AI"=w6290:refnum<k21>, "E_AI"=w6291:errorcluster)
                                n2803 = for {
                                tunnel: w6301 -> [w6306] mode=indexing
                                tunnel: w6300 -> [w6305] mode=indexing
                                tunnel: [w6304] -> w6296 mode=indexing
                                n2804 = call <vilib>:"DAQmx Stop Task.vi"("task/channels in"=w6306, "error in"=w6305) -> ("task out"=w6307:refnum<k21>, "error out"=w6308:errorcluster)  [unwired: 12 in]
                                n2805 = call <vilib>:"DAQmx Clear Task.vi"("task in"=w6307, "error in"=w6308) -> ("error out"=w6304:errorcluster)  [unwired: 13 in]
                                }
                                n2806 = call <vilib>:"DAQmx Stop Task.vi"("task/channels in"=w6290, "error in"=w6291) -> ("task out"=w6287:refnum<k21>, "error out"=w6286:errorcluster)  [unwired: 12 in]
                                n2807 = call <vilib>:"DAQmx Clear Task.vi"("task in"=w6287, "error in"=w6286) -> ("error out"=w6285:errorcluster)  [unwired: 13 in]
                                n2808 = call "tempconfigAO.vi"("command"="get") -> ("Temp Config out"=w6297:T28)  [unwired: 1 in]
                                n2809 = Bundle By Name(cluster=w6297, "E_AO"=w6296) -> (w6295:T28)
                                n2810 = call "tempconfigAI.vi"("command"="get") -> ("Temp Config out"=w6293:T29)  [unwired: 1 in]
                                n2811 = Bundle By Name(cluster=w6293, "E_AI"=w6285) -> (w6284:T29)
                                n2812 = call "tempconfigAO.vi"("Temp Config in"=w6295, "command"="set") -> ()  [unwired: 1 out]
                                n2813 = call "tempconfigAI.vi"("Temp Config in"=w6284, "command"="set") -> ()  [unwired: 1 out]
                                }
                              }
                              n2814 = call "allAI-temp.vi"("command"=enum16{"get", "set", "clear", "append"}."get") -> ("array out"=w6267:sgl[][])  [unwired: 3 in, 1 out]
                              n2815 = call "tempconfigAI.vi"("command"="get") -> ("Temp Config out"=w6279:T29)  [unwired: 1 in]
                              n2816 = call "tempconfigAI.vi"("command"="get") -> ("Temp Config out"=w6281:T29)  [unwired: 1 in]
                              n2817 = Unbundle By Name(w6279) -> ("header"=w6277:dbl[])
                              n2818 = Unbundle By Name(w6281) -> ("header"=w6283:dbl[])
                              n2819 = Index Array(array=w6267, index (row) #1=1 ("index (row)"), index (row) #2=0 ("index (row)")) -> (element #1=w6265:sgl[], element #2=w6264:sgl[])  [unwired: 2 in]
                              n2820 = local read "OCgain"() -> (w6271:sgl)
                              n2821 = call "Unscaledtoscaled.vi"("Unscaled Data"=w6265, "Header Information"=w6277) -> ("Array"=w6276:sgl[])  [unwired: 1 in]
                              n2822 = call "Unscaledtoscaled.vi"("Unscaled Data"=w6264, "Header Information"=w6283) -> ("Array"=w6280:sgl[])  [unwired: 1 in]
                              n2823 = Multiply(x=w6276, y=0.1) -> (x*y=w6273:dbl[])
                              n2824 = Divide(x=w6280, y=w6271) -> (x/y=w6272:sgl[])
                              n2825 = Build Array(w6273, w6272) -> (w6275:dbl[][])
                              n2826 = Multiply(x=w6275, y=1000.0) -> (x*y=w6262:dbl[][])
                              n2827 = local write "Patch readout"(w6262) -> ()
                            }
                            frame #4 {
                              n2828 = case shown="True" w6310 {
                                tunnel: w6309 -> [_ w6311]
                                frame False {
                                }
                                frame True {
                                n2829 = call "patchparameters.vi"("command"="get") -> ("Params out"=w6315:T16)  [unwired: 1 in]
                                n2830 = Unbundle By Name(w6315) -> ("holdon"=w6314:bool, "Vhold (mV)"=w6313:sgl, "CC_icg (pA/mv)"=w6321:sgl, "CC"=w6319:bool, "VC_icg (mV/mV)"=w6320:sgl)
                                n2831 = Select(t=w6321, s=w6319, f=w6320) -> (s? t:f=w6322:sgl)
                                n2832 = To Single Precision Float(number=0.001 ("y")) -> (single precision float=w6323:sgl)
                                n2833 = Compound Arithmetic op=MULTIPLY(w6313, w6322, w6323) -> (w6317:sgl)
                                n2834 = case shown="True" w6314 {
                                tunnel: w6317 -> [_ w6328]
                                tunnel: [0.0 w6328] -> w6312
                                frame False {
                                }
                                frame True {
                                }
                                }
                                n2835 = flat-sequence {
                                tunnel: w6311 -> [w6324]
                                tunnel: w6312 -> [w6326]
                                tunnel: w6311 -> [w6325]
                                frame #0 {
                                n2836 = call "prepAI_sealtest.vi"("samples per channel"=w6324) -> ()  [unwired: 2 in]
                                }
                                frame #1 {
                                n2837 = call "prepAO_sealtest.vi"("Vhold"=w6326, "samples per channel"=w6325) -> ()  [unwired: 1 in]
                                }
                                }
                                }
                              }
                            }
                            frame #5 {
                              n2838 = case shown="True" w6329 {
                                frame False {
                                }
                                frame True {
                                n2839 = stacked-sequence {
                                frame #0 {
                                n2840 = call "tempconfigAO.vi"("command"="get") -> ("Temp Config out"=w6336:T28)  [unwired: 1 in]
                                n2841 = Unbundle By Name(w6336) -> ("AO"=w6335:refnum<k21>[], "E_AO"=w6334:errorcluster[])
                                n2842 = for {
                                tunnel: w6335 -> [w6343] mode=indexing
                                tunnel: w6334 -> [w6342] mode=indexing
                                tunnel: [w6341] -> w6332 mode=indexing
                                tunnel: [w6340] -> w6331 mode=indexing
                                n2843 = call <vilib>:"DAQmx Start Task.vi"("task/channels in"=w6343, "error in"=w6342) -> ("task out"=w6341:refnum<k21>, "error out"=w6340:errorcluster)  [unwired: 12 in]
                                }
                                n2844 = call "tempconfigAO.vi"("command"="get") -> ("Temp Config out"=w6333:T28)  [unwired: 1 in]
                                n2845 = Bundle By Name(cluster=w6333, "AO"=w6332, "E_AO"=w6331) -> (w6330:T28)
                                n2846 = call "tempconfigAO.vi"("Temp Config in"=w6330, "command"="set") -> ()  [unwired: 1 out]
                                }
                                frame #1 {
                                n2847 = call "tempconfigAI.vi"("command"="get") -> ("Temp Config out"=w6345:T29)  [unwired: 1 in]
                                n2848 = Unbundle By Name(w6345) -> ("AI"=w6350:refnum<k21>, "E_AI"=w6351:errorcluster)
                                n2849 = call <vilib>:"DAQmx Start Task.vi"("task/channels in"=w6350, "error in"=w6351) -> ("task out"=w6352:refnum<k21>, "error out"=w6353:errorcluster)  [unwired: 12 in]
                                n2850 = call "tempconfigAI.vi"("command"="get") -> ("Temp Config out"=w6347:T29)  [unwired: 1 in]
                                n2851 = Bundle By Name(cluster=w6347, "AI"=w6352, "E_AI"=w6353) -> (w6349:T29)
                                n2852 = call "tempconfigAI.vi"("Temp Config in"=w6349, "command"="set") -> ()  [unwired: 1 out]
                                }
                                }
                                }
                              }
                            }
                          }
                        }
                        frame True {
                        }
                      }
                      n2853 = local read "readpatch"() -> (w6227:bool)
                      n2854 = Not(x=w6227) -> (.not. x?=w6226:bool)
                    }
                  }
                  frame #4 {
                    n2855 = call "tempconfigAO.vi"("command"="get") -> ("Temp Config out"=w6379:T28)  [unwired: 1 in]
                    n2856 = Unbundle By Name(w6379) -> ("AO"=w6378:refnum<k21>[], "E_AO"=w6377:errorcluster[])
                    n2857 = call "configuration.vi"("command"="get") -> ("config out"=w6360:T14)  [unwired: 2 in, 1 out]
                    n2858 = call "tempconfigAI.vi"("command"="get") -> ("Temp Config out"=w6366:T29)  [unwired: 1 in]
                    n2859 = Unbundle By Name(w6360) -> ("Device 1 sampleclock out"=w6357:tag, "Device 1 Starttrigger out"=w6356:tag)
                    n2860 = Unbundle By Name(w6366) -> ("AI"=w6367:refnum<k21>, "E_AI"=w6368:errorcluster)
                    n2861 = for {
                      tunnel: w6378 -> [w6383] mode=indexing
                      tunnel: w6377 -> [w6382] mode=indexing
                      tunnel: [w6381] -> w6373 mode=indexing
                      n2862 = call <vilib>:"DAQmx Stop Task.vi"("task/channels in"=w6383, "error in"=w6382) -> ("task out"=w6384:refnum<k21>, "error out"=w6385:errorcluster)  [unwired: 12 in]
                      n2863 = call <vilib>:"DAQmx Clear Task.vi"("task in"=w6384, "error in"=w6385) -> ("error out"=w6381:errorcluster)  [unwired: 13 in]
                    }
                    n2864 = call <vilib>:"DAQmx Stop Task.vi"("task/channels in"=w6367, "error in"=w6368) -> ("task out"=w6364:refnum<k21>, "error out"=w6363:errorcluster)  [unwired: 12 in]
                    n2865 = call <vilib>:"DAQmx Disconnect Terminals.vi"("source terminal"=tag "/Dev1/ai/SampleClock", "destination terminal"=w6357) -> ("error out"=w6354:errorcluster)  [unwired: 13 in]
                    n2866 = call <vilib>:"DAQmx Clear Task.vi"("task in"=w6364, "error in"=w6363) -> ("error out"=w6362:errorcluster)  [unwired: 13 in]
                    n2867 = call "tempconfigAO.vi"("command"="get") -> ("Temp Config out"=w6374:T28)  [unwired: 1 in]
                    n2868 = Bundle By Name(cluster=w6374, "E_AO"=w6373) -> (w6372:T28)
                    n2869 = call "tempconfigAI.vi"("command"="get") -> ("Temp Config out"=w6370:T29)  [unwired: 1 in]
                    n2870 = Bundle By Name(cluster=w6370, "E_AI"=w6362) -> (w6361:T29)
                    n2871 = call "tempconfigAO.vi"("Temp Config in"=w6372, "command"="set") -> ()  [unwired: 1 out]
                    n2872 = call <vilib>:"DAQmx Disconnect Terminals.vi"("source terminal"=tag "/Dev1/ai/StartTrigger", "destination terminal"=w6356, "error in"=w6354) -> ()  [unwired: 12 in, 1 out]
                    n2873 = call "tempconfigAI.vi"("Temp Config in"=w6361, "command"="set") -> ()  [unwired: 1 out]
                  }
                  frame #5 {
                    w6388 = T24 4 items=["no dialog", "OK message", "continue or stop message", "OK message + warnings", "continue/stop + warnings"] ("type of dialog (OK msg:1)")
                    n2874 = call "displayerrors.vi"() -> ("error IO"=w6387:errorcluster)
                    n2875 = call "zeropatch.vi"() -> ()  [unwired: 12 in]
                    n2876 = call <vilib>:"Simple Error Handler.vi"("type of dialog (OK msg:1)"=w6388, "error in (no error)"=w6387) -> ("error out"=w6386:errorcluster)  [unwired: 3 in, 4 out]
                    n2877 = call <vilib>:"Clear Errors.vi"("error in (no error)"=w6386) -> ()  [unwired: 5 in, 2 out]
                  }
                }
              }
            }
          }
          event "Current Clamp": Value Change {
            n2878 = event-data() -> ()  [unwired: 1 in, 6 out]
            n2879 = local read "Current Clamp"() -> (w6393:bool)
            n2880 = property on="Vholding (mV)" class="DigNum (strict)"("Caption.Text"="Ihold (pA)") -> ()  [unwired: 2 in, 2 out]
            n2881 = Not(x=w6393) -> (.not. x?=w6392:bool)
            n2882 = property on="Voltage Clamp" class="Bool (strict)"("Value"=w6392) -> ()  [unwired: 2 in, 2 out]
            n2883 = One Button Dialog(message="Have you switched the HEKA to CC and changed the external input cable?", button name ("OK")="Ok") -> ()  [unwired: 1 out]
          }
          event "Voltage Clamp": Value Change {
            n2884 = event-data() -> ()  [unwired: 1 in, 6 out]
            n2885 = local read "Voltage Clamp"() -> (w6398:bool)
            n2886 = Not(x=w6398) -> (.not. x?=w6397:bool)
            n2887 = property on="Current Clamp" class="Bool (strict)"("Value"=w6397) -> ()  [unwired: 2 in, 2 out]
            n2888 = One Button Dialog(message="Have you switched the HEKA to VC and changed the external input cable?", button name ("OK")="Ok") -> ()  [unwired: 1 out]
            n2889 = property on="Vholding (mV)" class="DigNum (strict)"("Caption.Text"="Vhold (mV)") -> ()  [unwired: 2 in, 2 out]
          }
          event "OCgain": Value Change {
            n2890 = event-data() -> ()  [unwired: 1 in, 6 out]
            n2891 = local read "OCgain"() -> (w6401:sgl)
            n2892 = Less?(x=w6401, y=0.3) -> (x < y?=w6399:bool)
            n2893 = case shown="True" w6399 {
              frame False {
                w6402 = 10.0 items=["0.1"=10.0, "10"=0.1] ("CC_ICgain")
                n2894 = local write "CC_ICgain"(w6402) -> ()
              }
              frame True {
                w6403 = 0.1 items=["0.1"=10.0, "10"=0.1] ("CC_ICgain")
                n2895 = local write "CC_ICgain"(w6403) -> ()
              }
            }
          }
          event "holdon": Value Change {
            n2896 = event-data() -> ()  [unwired: 1 in, 6 out]
            n2897 = stacked-sequence {
              frame #0 {
                n2898 = local read "Vholding (mV)"() -> (w6407:sgl)
                n2899 = local read "holdon"() -> (w6404:bool)
                n2900 = call "patchparameters.vi"("command"="get") -> ("Params out"=w6408:T16)  [unwired: 1 in]
                n2901 = Bundle By Name(cluster=w6408, "Vhold (mV)"=w6407, "holdon"=w6404) -> (w6405:T16)
                n2902 = call "patchparameters.vi"("Params in"=w6405, "command"="set") -> ()  [unwired: 1 out]
              }
              frame #1 {
                n2903 = call "zeropatch.vi"() -> ()  [unwired: 12 in]
              }
            }
          }
          event "Vholding (mV)": Value Change {
            n2904 = event-data() -> ()  [unwired: 1 in, 6 out]
            n2905 = local read "holdon"() -> (w6410:bool)
            n2906 = case shown="True" w6410 {
              frame False {
              }
              frame True {
                n2907 = stacked-sequence {
                  frame #0 {
                    n2908 = local read "Vholding (mV)"() -> (w6413:sgl)
                    n2909 = local read "holdon"() -> (w6414:bool)
                    n2910 = call "patchparameters.vi"("command"="get") -> ("Params out"=w6415:T16)  [unwired: 1 in]
                    n2911 = Bundle By Name(cluster=w6415, "Vhold (mV)"=w6413, "holdon"=w6414) -> (w6411:T16)
                    n2912 = call "patchparameters.vi"("Params in"=w6411, "command"="set") -> ()  [unwired: 1 out]
                  }
                  frame #1 {
                    n2913 = call "zeropatch.vi"() -> ()  [unwired: 12 in]
                  }
                }
              }
            }
          }
          event "AI channels": Value Change {
            n2914 = event-data() -> ()  [unwired: 1 in, 6 out]
            n2915 = local read "CI channels"() -> (w6424:i32[])
            n2916 = local read "AI channels"() -> (w6425:i32[])
            n2917 = call "configuration.vi"("command"="get") -> ("config out"=w6419:T14)  [unwired: 2 in, 1 out]
            n2918 = Unbundle By Name(w6419) -> ("CI names"=w6420:string[], "AI names"=w6421:string[])
            n2919 = for {
              tunnel: w6424 -> [w6430] mode=indexing
              tunnel: w6420 -> [w6431]
              tunnel: [w6429] -> w6422 mode=indexing
              n2920 = Index Array(array=w6431, index=w6430) -> (element=w6429:string)
            }
            n2921 = for {
              tunnel: w6425 -> [w6427] mode=indexing
              tunnel: w6421 -> [w6428]
              tunnel: [w6426] -> w6423 mode=indexing
              n2922 = Index Array(array=w6428, index=w6427) -> (element=w6426:string)
            }
            n2923 = Build Array (concatenate)(w6422, w6423) -> (w6417:string[])
            n2924 = property on="image1list" class="Ring (strict)"("Strings []"=w6417) -> ()  [unwired: 2 in, 2 out]
            n2925 = property on="image2list" class="Ring (strict)"("Strings []"=w6417) -> ()  [unwired: 2 in, 2 out]
            n2926 = property on="image1list chA" class="Ring (strict)"("Strings []"=w6417) -> ()  [unwired: 2 in, 2 out]
            n2927 = property on="image1list chB" class="Ring (strict)"("Strings []"=w6417) -> ()  [unwired: 2 in, 2 out]
          }
          event "CI channels": Value Change {
            n2928 = event-data() -> ()  [unwired: 1 in, 6 out]
            n2929 = local read "CI channels"() -> (w6439:i32[])
            n2930 = local read "AI channels"() -> (w6440:i32[])
            n2931 = call "configuration.vi"("command"="get") -> ("config out"=w6434:T14)  [unwired: 2 in, 1 out]
            n2932 = Unbundle By Name(w6434) -> ("CI names"=w6435:string[], "AI names"=w6436:string[])
            n2933 = for {
              tunnel: w6439 -> [w6445] mode=indexing
              tunnel: w6435 -> [w6446]
              tunnel: [w6444] -> w6437 mode=indexing
              n2934 = Index Array(array=w6446, index=w6445) -> (element=w6444:string)
            }
            n2935 = for {
              tunnel: w6440 -> [w6442] mode=indexing
              tunnel: w6436 -> [w6443]
              tunnel: [w6441] -> w6438 mode=indexing
              n2936 = Index Array(array=w6443, index=w6442) -> (element=w6441:string)
            }
            n2937 = Build Array (concatenate)(w6437, w6438) -> (w6432:string[])
            n2938 = property on="image1list" class="Ring (strict)"("Strings []"=w6432) -> ()  [unwired: 2 in, 2 out]
            n2939 = property on="image2list" class="Ring (strict)"("Strings []"=w6432) -> ()  [unwired: 2 in, 2 out]
            n2940 = property on="image1list chA" class="Ring (strict)"("Strings []"=w6432) -> ()  [unwired: 2 in, 2 out]
            n2941 = property on="image1list chB" class="Ring (strict)"("Strings []"=w6432) -> ()  [unwired: 2 in, 2 out]
          }
          event "setdatdir": Value Change {
            n2942 = event-data() -> ()  [unwired: 1 in, 5 out]
            n2943 = case shown="True" "setdatdir" {
              frame False {
              }
              frame True {
                n2944 = stacked-sequence {
                  frame #0 {
                    n2945 = local read "data dir"() -> (w6448:path)
                    n2946 = call "File Dialog"("start path"=w6448, "prompt"="Please select data directory...") -> ("selected path"=w6450:path, "cancelled"=w6449:bool, "error out"=w6451:errorcluster)  [unwired: 10 in, 1 out]
                    n2947 = case shown="False" w6449 {
                      tunnel: w6450 -> [w6459 _]
                      tunnel: w6451 -> [w6456 w6462]
                      tunnel: [w6454 w6462] -> w6453
                      frame False {
                        n2948 = local write "data dir"(w6459) -> ()
                        n2949 = call "configuration.vi"("error in"=w6456, "command"="get") -> ("Error out"=w6455:errorcluster, "config out"=w6461:T14)  [unwired: 1 in]
                        n2950 = Bundle By Name(cluster=w6461, "master data dir"=w6459) -> (w6460:T14)
                        n2951 = call "configuration.vi"("error in"=w6455, "config in"=w6460, "command"="set") -> ("Error out"=w6454:errorcluster)  [unwired: 1 out]
                      }
                      frame True {
                      }
                    }
                    n2952 = local write "status"(w6453) -> ()
                  }
                  frame #1 {
                    n2953 = property on="setdatdir" class="Bool (strict)"("Value"=FALSE ("setdatdir")) -> ()  [unwired: 2 in, 2 out]
                  }
                }
              }
            }
          }
          event "Shutter": Value Change {
            n2954 = event-data() -> ()  [unwired: 1 in, 5 out]
            n2955 = local read "Auto Shutter Channels"() -> (w6464:i32[])
            n2956 = case shown="True" "Shutter" {
              tunnel: w6464 -> [w6466 w6468]
              frame False {
                n2957 = call "shuttercontrol_multi.vi"("Autoshutter Chans"=w6466, "command"="close") -> ()  [unwired: 1 in, 1 out]
              }
              frame True {
                n2958 = call "shuttercontrol_multi.vi"("Autoshutter Chans"=w6468, "command"="open") -> ()  [unwired: 1 in, 1 out]
              }
            }
          }
          event "ROI": Value Change {
            n2959 = event-data() -> ()  [unwired: 1 in, 5 out]
            n2960 = local read "ROI"() -> (w6470:bool)
            n2961 = case shown="True" w6470 {
              frame False {
              }
              frame True {
                n2962 = stacked-sequence {
                  frame #0 {
                    n2963 = local read "Square pixels"() -> (w6487:bool)
